vi "Import.vi"(8 "error in":errorcluster, 11 "CSV Path":path=path "C:/Users/Administrator/Desktop/FPGA Wizard/Exported IO.csv") -> (0 "error out":errorcluster, 3 "FPGA Settings":T1[](array[typedef]))   [LabVIEW 2025, in "Project.lvclass"]
doc: "Read CSV String and convert to structured cluster."
uses:
  Project.lvclass
  FPGA Settings.ctl
  Module/Module/Module Settings.ctl
  Signal/Signal/Signal Settings.ctl
  Signal/Signal/Signal.lvclass
  Module/Module/Module.lvclass
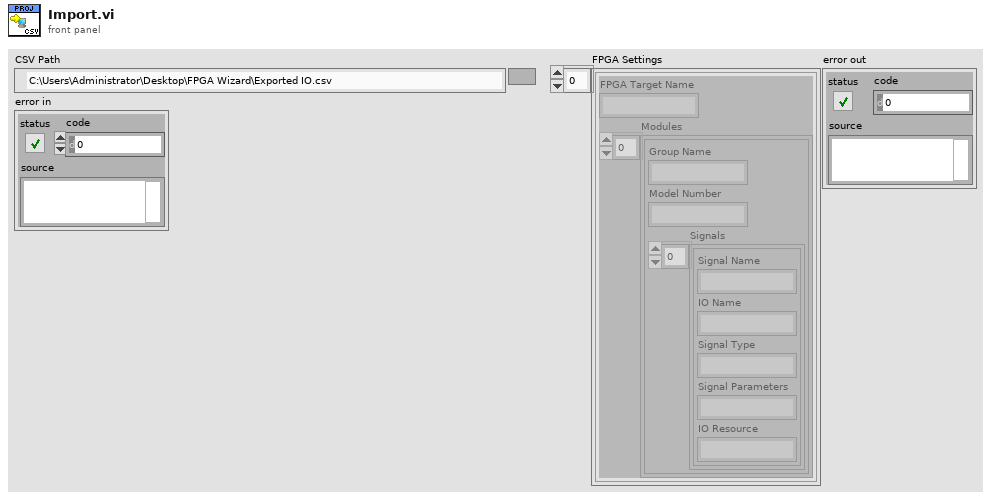
[diagram p1: front panel]
types:
  T1 = typedef "Project.lvclass/FPGA Settings.ctl" = cluster{"FPGA Target Name":string, "Modules":T2[]}
  T2 = typedef "Module.lvclass/Module Settings.ctl" = cluster{"Group Name":string, "Model Number":string, "Signals":T3[]}
  T3 = typedef "Signal.lvclass/Signal Settings.ctl" = cluster{"Signal Name":string, "IO Name":string, "Signal Type":string, "Signal Parameters":string, "IO Resource":string}
  T4 = enum16{"open", "replace", "create", "open or create", "replace or create", "replace or create with confirmation"}
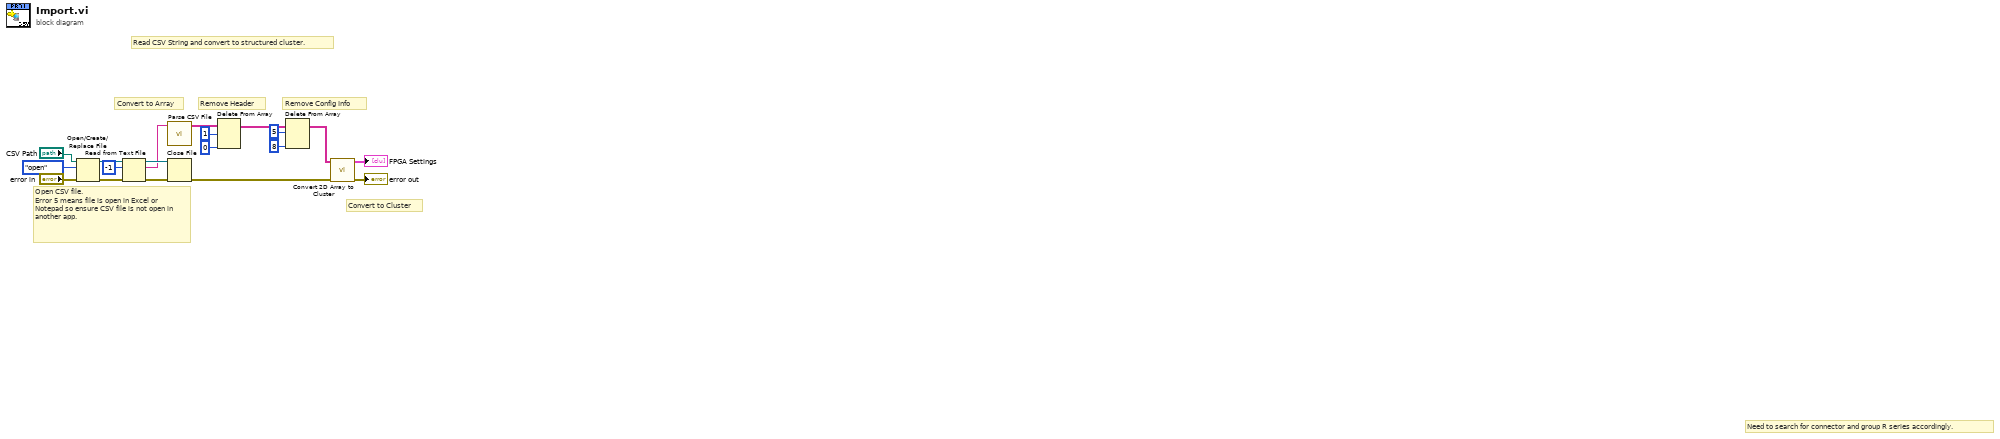
[diagram p0: block diagram]
diagram:
  # "Read CSV String and convert to structured cluster."
  # "Convert to Cluster"
  # "Convert to Array"
  # "Remove Config Info"
  # "Remove Header"
  # "Open CSV file.\nError 5 means file is open in Excel or Notepad so ensure CSV file is not open in another app."
  # "Need to search for connector and group R series accordingly."
  n1 = Open/Create/Replace File(file path (use dialog)="CSV Path", error in="error in", operation (0:open)=T4."open") -> (refnum out=w19:refnum<file>, error out=w16:errorcluster)  [unwired: 3 in, 1 out]
  n2 = Read from Text File(file (use dialog)=w19, count=-1, error in=w16) -> (refnum out=w18:refnum<file>, text=w7:string, error out=w17:errorcluster)  [unwired: 1 in, 1 out]
  n3 = call "Parse CSV File.vi"("String"=w7) -> ("Array"=w6:string[][])  [unwired: 10 in]
  n4 = Close File(refnum=w18, error in=w17) -> (error out=w10:errorcluster)  [unwired: 1 out]
  n5 = Delete From Array(array=w6, length=1, index (row)=0) -> (array with subset deleted=w4:string[][])  [unwired: 1 in, 1 out]
  n6 = Delete From Array(array=w4, length=5, index (col)=8 ("disabled index (col)")) -> (array with subset deleted=w3:string[][])  [unwired: 1 in, 1 out]
  n7 = call "Convert 2D Array to Cluster.vi"("error in (no error)"=w10, "Array in"=w3) -> ("error out"=→"error out":errorcluster, "Array out"=→"FPGA Settings":T1[])  [unwired: 8 in]
